vi "LIDAR Data Acquisition.vi"() -> (1 "LIDAR Data":T1)   [LabVIEW 2009]
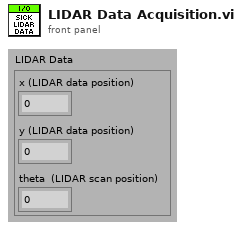
[diagram p1: front panel]
types:
  T1 = cluster{"x (LIDAR data position)":i16, "y (LIDAR data position) ":i16, "theta  (LIDAR scan position)":u8}
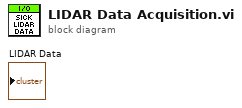
[diagram p0: block diagram]
diagram:
